vi "Count Module Usage in Connections.vi"(8 "error in (no error)":errorcluster, 10 "Module path":string, 11 "All State Configurations":cluster{"State Configurations":T1}[](array[cluster])) -> (0 "error out":errorcluster, 3 "Number of Usages":i32)   [LabVIEW 2017, in "Routing and Faulting System Explorer.lvlib"]
uses:
  Routing and Faulting System Explorer.lvlib
  Shared/Channel States.ctl
  Shared/Routing State.ctl
  Shared/Connection.ctl
  Shared/Routing and Faulting Shared.lvlib
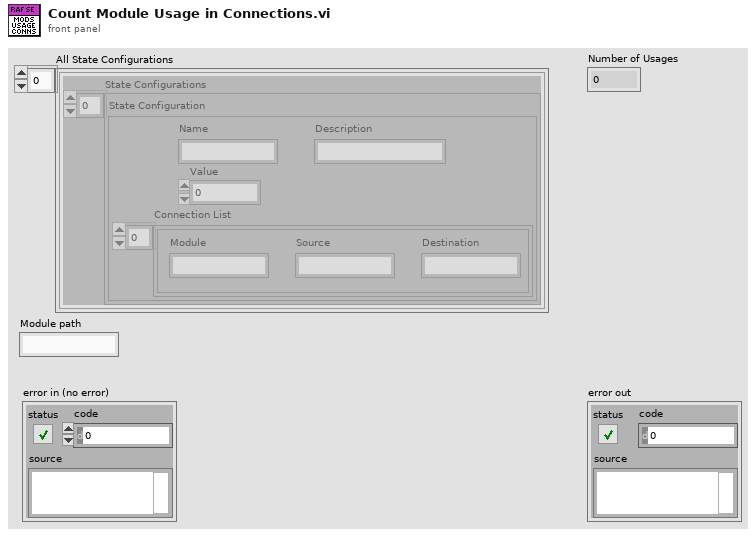
[diagram p1: front panel]
types:
  T1 = typedef "Routing and Faulting Shared.lvlib/Channel States.ctl" = T2[]
  T2 = typedef "Routing and Faulting Shared.lvlib/Routing State.ctl" = cluster{"Name":string, "Description":string, "Value":i32, "Connection List":T3[]}
  T3 = typedef "Routing and Faulting Shared.lvlib/Connection.ctl" = cluster{"Module":string, "Source":string, "Destination":string}
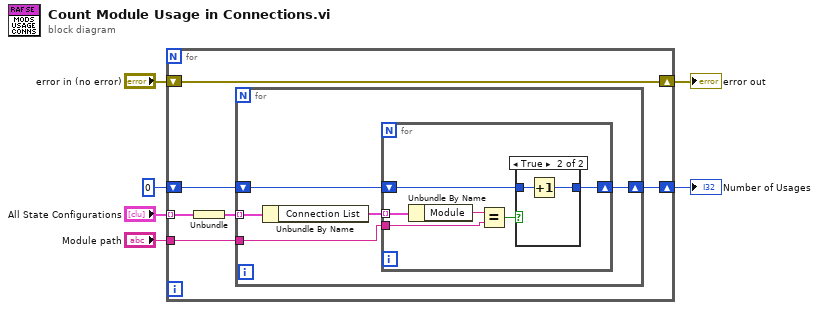
[diagram p0: block diagram]
diagram:
  n1 = for {
    tunnel: "All State Configurations" -> [w12] mode=indexing
    tunnel: "Module path" -> [w10]
    shift-right: [w8] -> w4
    shift-left: 0 -> [w9]
    shift-right: [w7] -> w6
    shift-left: "error in (no error)" -> [w7]
    n2 = Unbundle(w12) -> ("State Configurations"=w11:T1)
    n3 = for {
      tunnel: w11 -> [w17] mode=indexing
      tunnel: w10 -> [w15]
      shift-right: [w13] -> w8
      shift-left: w9 -> [w14]
      n4 = Unbundle By Name(w17) -> ("Connection List"=w16:T3[])
      n5 = for {
        tunnel: w16 -> [w23] mode=indexing
        tunnel: w15 -> [w21]
        shift-right: [w18] -> w13
        shift-left: w14 -> [w19]
        n6 = Unbundle By Name(w23) -> ("Module"=w22:string)
        n7 = Equal?(x=w22, y=w21) -> (x = y?=w20:bool)
        n8 = case shown="True" w20 {
          tunnel: w19 -> [w24 w26]
          tunnel: [w24 w25] -> w18
          frame False {
          }
          frame True {
            n9 = Increment(x=w26) -> (x+1=w25:i32)
          }
        }
      }
    }
  }
  "error out" <- w6
  "Number of Usages" <- w4
